vi "Remote PC - Client_DUT X.vi"(0 "IP Address":string="localhost", 2 "Flow Contorl":enum16{"Connect", "Read", "Write", "Close"}(ring)=enum."Write", 5 "Log Path":path=path "D:/My Projects/MitraStar/wlan test lib - onsite - second round/Report SubVIs/DUT 1_9_09_38 AM 10_24_2013_Report.csv", 7 "Send Command":T1="Analyze Log", 9 "ServerTCPhandle":refnum<k5>, 11 "error in":errorcluster, 12 "Remote Sever Port (2800)":u16) -> (3 "status":bool, 4 "sn":string, 6 "TCPHandle":refnum<k5>, 8 "mac":string, 10 "Receive Message":string, 13 "ServerTCPhandle 2":refnum<k5>, 14 "status 2":bool, 15 "error out":errorcluster)   [LabVIEW 2012]
uses:
  TypeDef/Send Command Message.ctl
panel:
  out "concatenated string":string
  out "bytes written":i32=19538
  out "data out":string="DONE\r\n"
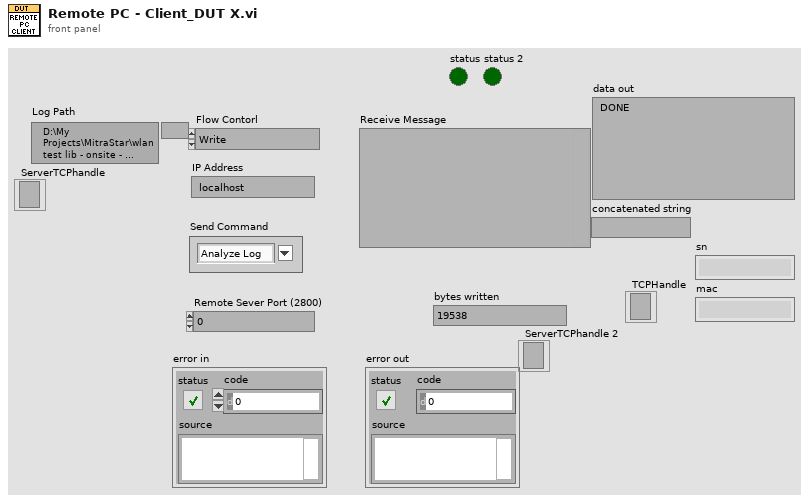
[diagram p1: front panel]
types:
  T1 = typedef "Send Command Message.ctl" = string
  T2 = enum16{"Standard", "Buffered", "CRLF", "Immediate"}
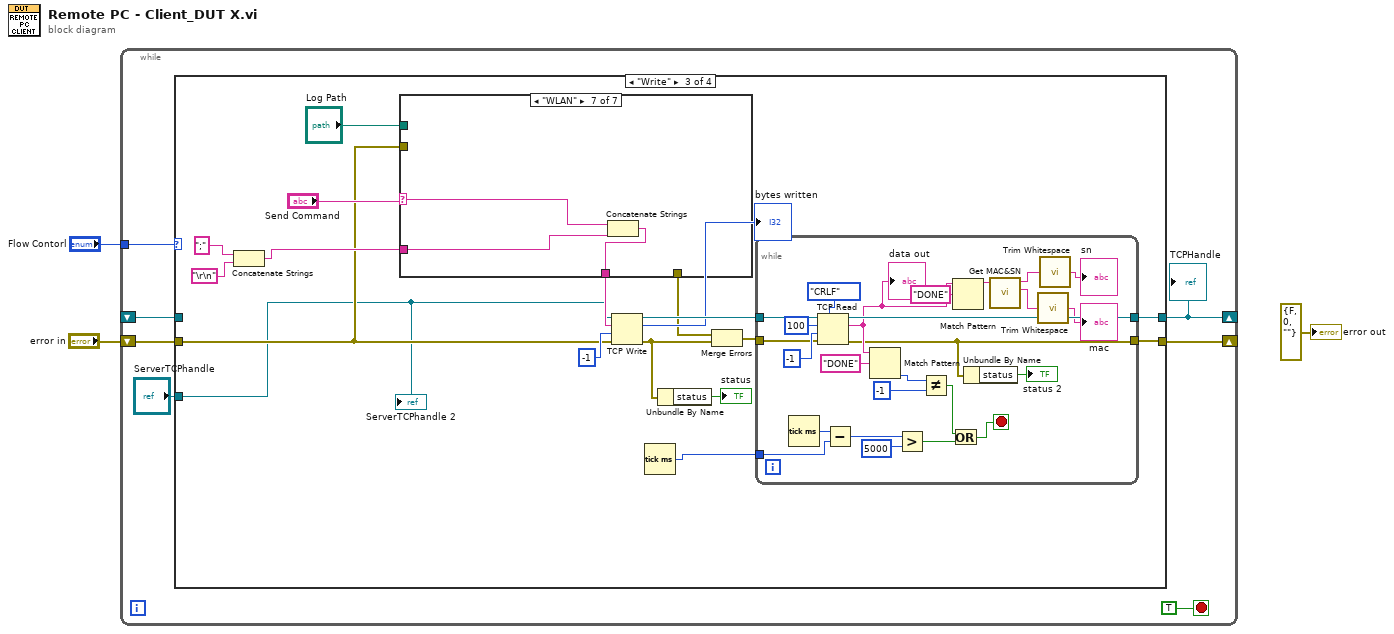
[diagram p0: block diagram]
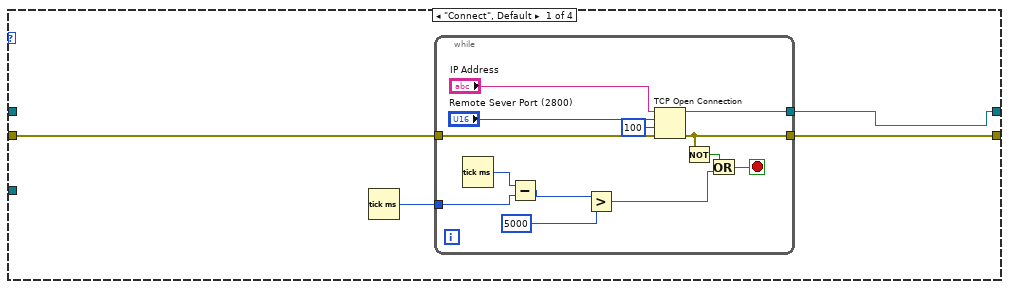
[diagram p2: hidden frame]
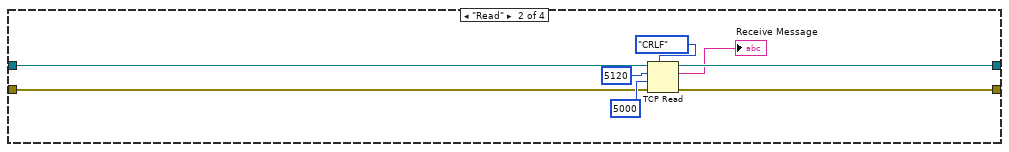
[diagram p3: hidden frame]
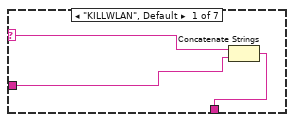
[diagram p4: hidden frame]
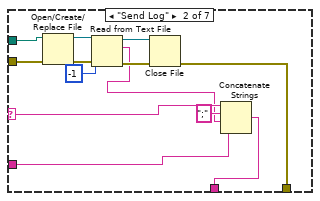
[diagram p5: hidden frame]
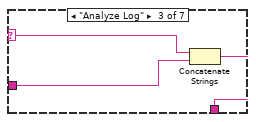
[diagram p6: hidden frame]
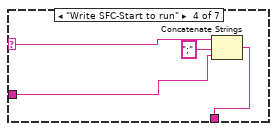
[diagram p7: hidden frame]
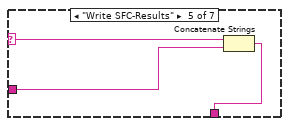
[diagram p8: hidden frame]
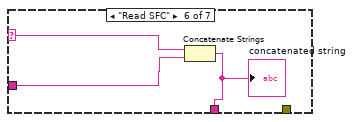
[diagram p9: hidden frame]
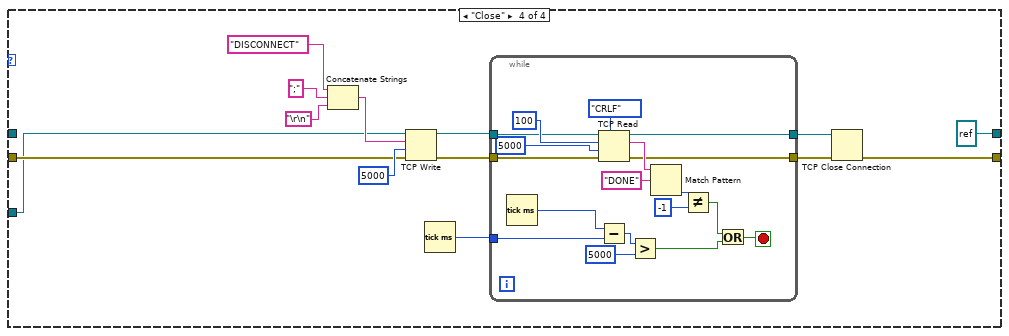
[diagram p10: hidden frame]
diagram:
  n1 = while {
    shift-right: [w8] -> _
    shift-left: "error in" -> [w9]
    shift-right: [w4] -> _
    shift-left: _ -> [w7]
    tunnel: "Flow Contorl" -> [w6]
    stop <- TRUE stop-if-true
    n2 = case shown="\"Write\"" w6 {
      tunnel: w9 -> [w14 w31 w41 w121]
      tunnel: [w13 w30 w50 w124] -> w8
      tunnel: [w11 w29 w51 refnum<k5> refnum ("connection ID")] -> w4
      tunnel: w7 -> [_ w32 _ _]
      tunnel: "ServerTCPhandle" -> [_ _ w38 w111]
      frame "Connect", Default {
        n3 = Tick Count (ms)() -> (millisecond timer value=w12:u32)
        n4 = while {
          tunnel: w14 -> [w25]
          tunnel: [w16] -> w13
          tunnel: [w24] -> w11
          tunnel: w12 -> [w21]
          stop <- w17 stop-if-true
          n5 = Tick Count (ms)() -> (millisecond timer value=w22:u32)
          n6 = Subtract(x=w22, y=w21) -> (x-y=w20:u32)
          n7 = Greater?(x=w20, y=u32 5000) -> (0:w18:bool)
          n8 = TCP Open Connection(address="IP Address", remote port or service name="Remote Sever Port (2800)", timeout ms (60000)=100, error in (no error)=w25) -> (connection ID=w24:refnum<k5>, error out=w16:errorcluster)  [unwired: 1 in]
          n9 = Not(x=w16) -> (.not. x?=w15:bool)
          n10 = Or(x=w15, y=w18) -> (x .or. y?=w17:bool)
        }
      }
      frame "Read" {
        n11 = TCP Read(connection ID=w32, bytes to read=5120, error in (no error)=w31, 7:T2."CRLF" ("mode (standard)"), 9:5000 ("timeout ms (25000)")) -> (connection ID out=w29:refnum<k5>, data out=→"Receive Message":string, error out=w30:errorcluster)
      }
      frame "Write" {
        n12 = Concatenate Strings(";", "\r\n") -> (w45:string)
        n13 = case shown="\"WLAN\"" "Send Command" {
          selector: "Send Command" -> [w56 w68 w72 w75 w79 w82 w85]
          tunnel: [w55 w69 w71 w76 w77 w81 w84] -> w48
          tunnel: w45 -> [w54 w66 w70 w73 w78 w80 w83]
          tunnel: "Log Path" -> [_ w60 _ _ _ _ _]
          tunnel: w41 -> [_ w59 _ _ _ _ _]
          tunnel: [_ w58 _ _ _ _ _] -> w39
          frame "KILLWLAN", Default {
            n14 = Concatenate Strings(w56, w54) -> (w55:string)
          }
          frame "Send Log" {
            n15 = Open/Create/Replace File(file path (use dialog)=w60, error in=w59) -> (refnum out=w63:refnum<file>, error out=w62:errorcluster)  [unwired: 4 in, 1 out]
            n16 = Read from Text File(file (use dialog)=w63, count=-1, error in=w62) -> (refnum out=w65:refnum<file>, text=w61:string, error out=w64:errorcluster)  [unwired: 1 in, 1 out]
            n17 = Close File(refnum=w65, error in=w64) -> (error out=w58:errorcluster)  [unwired: 1 out]
            n18 = Concatenate Strings(w68, ";" ("string"), w61, w66) -> (w69:string)
          }
          frame "Analyze Log" {
            n19 = Concatenate Strings(w72, w70) -> (w71:string)
          }
          frame "Write SFC-Start to run" {
            n20 = Concatenate Strings(w75, ";" ("string"), w73) -> (w76:string)
          }
          frame "Write SFC-Results" {
            n21 = Concatenate Strings(w79, w78) -> (w77:string)
          }
          frame "Read SFC" {
            n22 = Concatenate Strings(w82, w80) -> (w81:string)
            "concatenated string" <- w81
          }
          frame "WLAN" {
            n23 = Concatenate Strings(w85, w83) -> (w84:string)
          }
        }
        n24 = TCP Write(connection ID=w38, data in=w48, error in (no error)=w41, 9:-1 ("timeout ms (25000)")) -> (connection ID out=w52:refnum<k5>, bytes written=→"bytes written":i32, error out=w37:errorcluster)
        n25 = Tick Count (ms)() -> (millisecond timer value=w42:u32)
        n26 = Unbundle By Name(w37) -> ("status"=→"status":bool)
        n27 = Merge Errors(w39, w37) -> (w40:errorcluster)
        n28 = while {
          tunnel: [w104] -> w51
          tunnel: [w87] -> w50
          tunnel: w52 -> [w103]
          tunnel: w40 -> [w102]
          tunnel: w42 -> [w98]
          stop <- w93 stop-if-true
          n29 = Tick Count (ms)() -> (millisecond timer value=w99:u32)
          n30 = TCP Read(connection ID=w103, bytes to read=100, error in (no error)=w102, 7:T2."CRLF" ("mode (standard)"), 9:-1 ("timeout ms (25000)")) -> (connection ID out=w104:refnum<k5>, data out=w101:string, error out=w87:errorcluster)
          "data out" <- w101
          n31 = Subtract(x=w99, y=w98) -> (x-y=w97:u32)
          n32 = Match Pattern(string=w101, regular expression="DONE") -> (offset past match=w107:i32)  [unwired: 1 in, 3 out]
          n33 = Greater?(x=w97, y=u32 5000) -> (0:w95:bool)
          n34 = Not Equal?(x=w107, y=-1) -> (x != y?=w94:bool)
          n35 = Or(x=w94, y=w95) -> (x .or. y?=w93:bool)
          n36 = Match Pattern(string=w101, regular expression="DONE") -> (before substring=w92:string)  [unwired: 1 in, 3 out]
          n37 = Unbundle By Name(w87) -> ("status"=→"status 2":bool)
          n38 = call "Get MAC&SN.vi"("MAC&SN"=w92) -> ("mac"=w89:string, "sn"=w91:string)  [unwired: 8 in, 1 out]
          n39 = call <vilib>:"Trim Whitespace.vi"("string"=w89) -> ("trimmed string"=→"mac":string)  [unwired: 1 in]
          n40 = call <vilib>:"Trim Whitespace.vi"("string"=w91) -> ("trimmed string"=→"sn":string)  [unwired: 1 in]
        }
        "ServerTCPhandle 2" <- w38
      }
      frame "Close" {
        n41 = Concatenate Strings("DISCONNECT" ("data in"), ";", "\r\n") -> (w112:string)
        n42 = TCP Write(connection ID=w111, data in=w112, error in (no error)=w121, 9:5000 ("timeout ms (25000)")) -> (connection ID out=w117:refnum<k5>, error out=w116:errorcluster)  [unwired: 1 out]
        n43 = Tick Count (ms)() -> (millisecond timer value=w120:u32)
        n44 = while {
          tunnel: w120 -> [w134]
          tunnel: [w128] -> w119
          tunnel: [w127] -> w118
          tunnel: w117 -> [w126]
          tunnel: w116 -> [w125]
          stop <- w129 stop-if-true
          n45 = Tick Count (ms)() -> (millisecond timer value=w135:u32)
          n46 = TCP Read(connection ID=w126, bytes to read=100, error in (no error)=w125, 7:T2."CRLF" ("mode (standard)"), 9:5000 ("timeout ms (25000)")) -> (connection ID out=w128:refnum<k5>, data out=w140:string, error out=w127:errorcluster)
          n47 = Subtract(x=w135, y=w134) -> (x-y=w133:u32)
          n48 = Greater?(x=w133, y=u32 5000) -> (0:w130:bool)
          n49 = Match Pattern(string=w140, regular expression="DONE") -> (offset past match=w138:i32)  [unwired: 1 in, 3 out]
          n50 = Not Equal?(x=w138, y=-1) -> (x != y?=w131:bool)
          n51 = Or(x=w131, y=w130) -> (x .or. y?=w129:bool)
        }
        n52 = TCP Close Connection(connection ID=w119, error in (no error)=w118) -> (error out=w124:errorcluster)  [unwired: 1 in, 1 out]
      }
    }
    "TCPHandle" <- w4
  }
  "error out" <- errorcluster {"status"=FALSE, "code"=0, "source"=""} ("error out")
